vi "DSF.Engine.Sequencer Bundle.Set Plugin Timing.vi"(8 "error in (no error)":errorcluster, 10 "Plugin Timing":refnum<class "DSF.Engine.Timing.lvclass">, 11 "Sequencer Bundle in":refnum<class "DSF.Engine.Sequencer Bundle.lvclass">) -> (0 "error out":errorcluster, 3 "Sequencer Bundle out":refnum<class "DSF.Engine.Sequencer Bundle.lvclass">)   [LabVIEW 2016, in "DSF.Engine.lvlib" / "DSF.Engine.Sequencer Bundle.lvclass"]
uses:
  DSF.Engine.Sequencer Bundle.lvclass
  Timing/DSF.Engine.Timing.lvclass
  DSF.Engine.Sequencer Bundle.lvclass/DSF.Engine.Sequencer Bundle.ctl
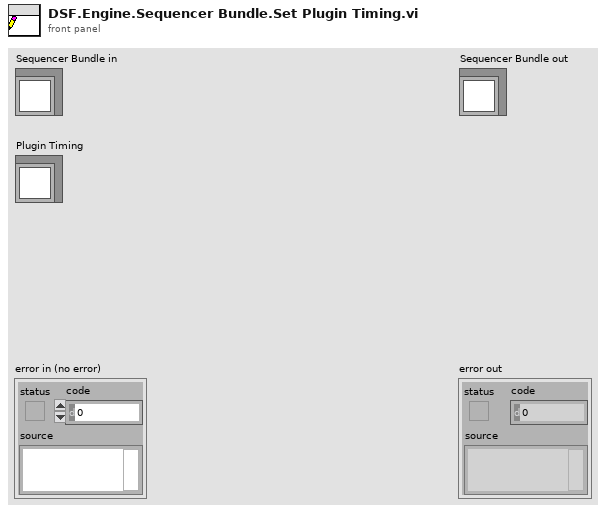
[diagram p1: front panel]
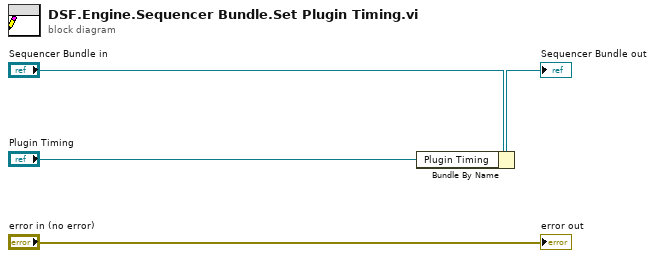
[diagram p0: block diagram]
diagram:
  n1 = Bundle By Name(cluster="Sequencer Bundle in", "Plugin Timing"="Plugin Timing") -> (→"Sequencer Bundle out":refnum<class "DSF.Engine.Sequencer Bundle.lvclass">)
  "error out" <- "error in (no error)"
